vi "BiPotentiostat.vi"(4 "RE_Segments":i16[](array[numeric])=[0, 0, 0], 5 "AI Count(uSec)":u32=5, 6 "TE_Segments":i16[](array[numeric])=[0, 0, 0], 7 "Segment_uSec":sgl[](array[numeric])=[0.0, 0.0, 0.0], 8 "BE_Segments":i16[](array[numeric])=[0, 0, 0], 9 "RE_Start":i16, 10 "TE_Start":i16, 11 "BE_Start":i16) -> ()   [LabVIEW 2019]
uses:
  <vilib>/rvi/Emulation/niFpgaGetClockAttributes.vi
  <vilib>/rvi/Emulation/niFpgaSctlEmulationGetInTimedLoop.vi
  <vilib>/rvi/Emulation/niFpgaEmulationReportErrorSimple.vi
  <vilib>/rvi/eio/common/nirviEmuTemplateMethod_errors.vi
  <vilib>/rvi/interface/RandomDataEmulation/niFpgaRandomDataHandleErrors.vi
  <vilib>/rvi/Emulation/niFpgaProcessEmulError.vi
  <vilib>/rvi/DataTransferAndStorage/Container/Common/niFpgaContainerExecOnDevCompGetState.vi
  <vilib>/rvi/Emulation/niFpgaEmulationIsFPGAContextNoSignature.vi
  <vilib>/rvi/errors/niFpgaSetErrorForExecOnDevCompSimple.vi
  <vilib>/rvi/eio/common/nirviEmuReportErrorAndStop.vi
  <vilib>/rvi/DataTransferAndStorage/Container/Common/niFpgaContainerGetUniqueNameForEmu.vi
  <vilib>/rvi/FIFO/Fifo_Resource/nirvififoEmulationSetSize.vi
  <vilib>/rvi/FIFO/Fifo_Resource/nirviFifoEmulationQueueMgr.vi
  <instcachedir>/0/nirviFifoEmulationQueueMgr_E5CAEC123FF24DC58D834DCA3CDAA9B5.lvgen/nirviFifoEmulationQueueMgr_E5CAEC123FF24DC58D834DCA3CDAA9B5_008.vi
  <vilib>/rvi/FIFO/Fifo_Resource/nirvififoEmulationDetermineInputValidOut.vi
  <vilib>/rvi/FIFO/Fifo_Resource/nirvififoEmulationCreateLock.vi
  <vilib>/rvi/FIFO/Fifo_Resource/nirvififoEmulationObtainLock.vi
  <vilib>/rvi/FIFO/Fifo_Resource/nirvififoEmulationReleaseLock.vi
  <vilib>/rvi/occurrence/nirviWaitOnOccurrenceBase.vi
  <vilib>/rvi/errors/nirviReportUnexpectedCaseInternalError.vi
  <vilib>/rvi/errors/nirviReportUnexpectedCaseInternalError (U32).vi
  <vilib>/Utility/error.llb/Clear Errors.vi
  <vilib>/rvi/Emulation/niFpgaCriticalErrorInLSC.vi
  <vilib>/eio/EIONode/EIONode.xnode
  <vilib>/rvi/DataTransferAndStorage/Container/XNode/niFpgaContainer.xnode
  <vilib>/rvi/interface/RandomDataEmulation/nirviRandomDataFpgaReadWriteTemplate.vi
  <vilib>/rvi/FIFO/Fifo_Resource/niFpgaFifoEmulationRefIn.vi
panel:
  out "Stop":bool
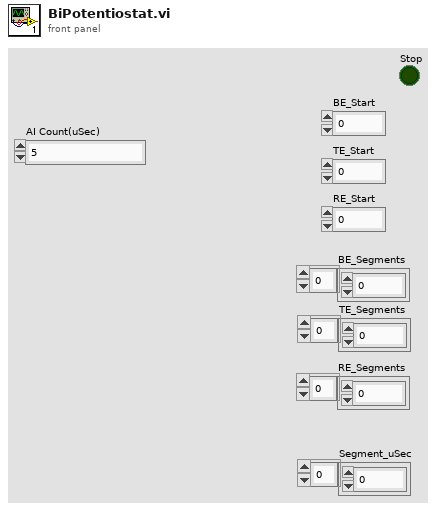
[diagram p1: front panel]
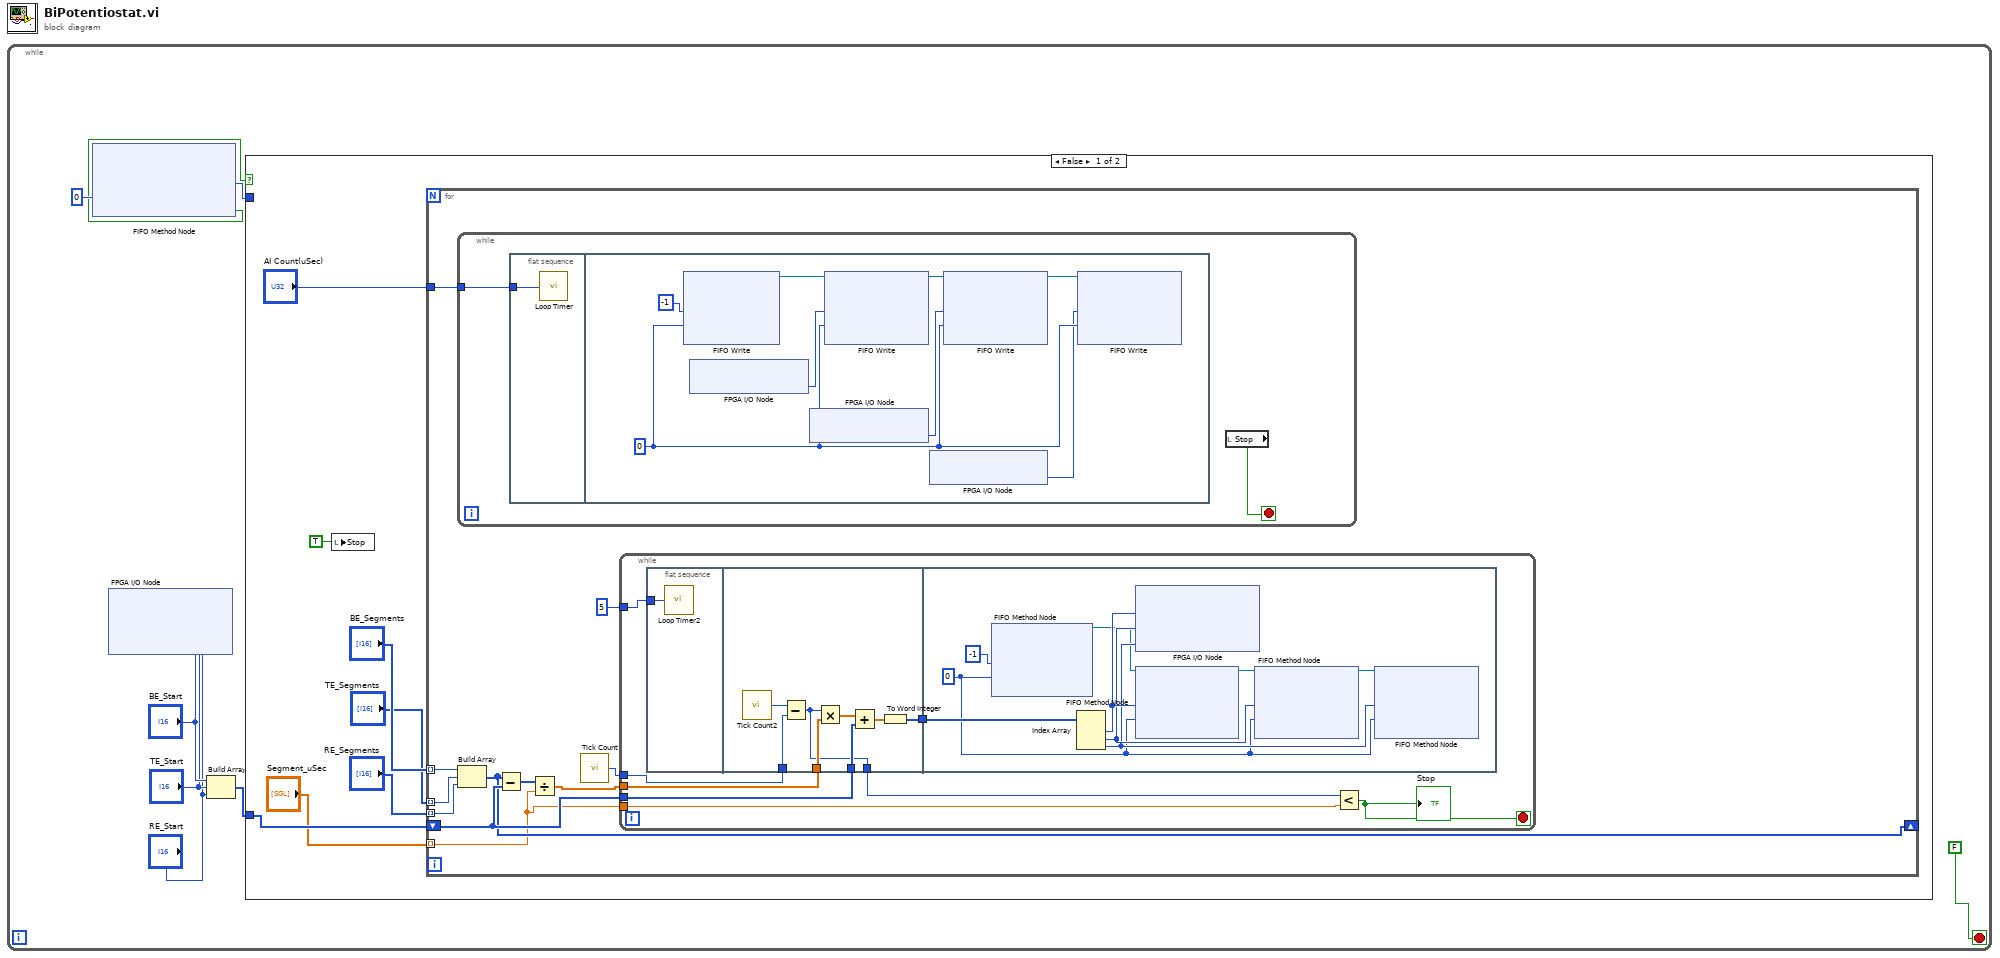
[diagram p0: block diagram]
diagram:
  n1 = while {
    stop <- FALSE stop-if-true
    n2 = xnode ("FIFO Method Node")("Timeout"=0) -> ("Element"=w6:i16, "Timed Out?"=w7:bool)  [unwired: 1 in, 1 out]
    n3 = xnode "FPGA I/O Node"("Connector0/AO0"="BE_Start", "Connector0/AO1"="TE_Start", "Connector0/AO2"="RE_Start") -> ()  [unwired: 3 in, 3 out]
    n4 = Build Array("BE_Start", "TE_Start", "RE_Start") -> (w1:i16[])
    n5 = case shown="False" w7 {
      tunnel: w6 -> [_ _]
      tunnel: w1 -> [w14 _]
      frame False {
        n6 = local write "Stop"(TRUE ("Stop")) -> ()
        n7 = for {
          tunnel: "AI Count(uSec)" -> [w26]
          shift-right: [w18] -> _
          shift-left: w14 -> [w19]
          tunnel: "Segment_uSec" -> [w16] mode=indexing
          tunnel: "BE_Segments" -> [w23] mode=indexing
          tunnel: "TE_Segments" -> [w22] mode=indexing
          tunnel: "RE_Segments" -> [w21] mode=indexing
          n8 = while {
            tunnel: w26 -> [w54]
            stop <- w53 stop-if-true
            n9 = flat-sequence {
              tunnel: w54 -> [w55]
              frame #0 {
                n10 = call "Loop Timer"("Count(uSec)"=w55) -> ()  [unwired: 1 out]
              }
              frame #1 {
                w60 = 0 ("Timeout")
                n11 = xnode ("FIFO Write")("Element"=i16 -1, "Timeout"=w60) -> ("FIFO Out"=w63:refnum<k21>)  [unwired: 1 in, 1 out]
                n12 = xnode "FPGA I/O Node"() -> ("Connector0/AI0"=w57:i16)  [unwired: 1 in, 1 out]
                n13 = xnode "FPGA I/O Node"() -> ("Connector0/AI1"=w58:i16)  [unwired: 1 in, 1 out]
                n14 = xnode ("FIFO Write")("Element"=w57, "Timeout"=w60, "FIFO In"=w63) -> ("FIFO Out"=w62:refnum<k21>)  [unwired: 1 out]
                n15 = xnode "FPGA I/O Node"() -> ("Connector0/AI2"=w59:i16)  [unwired: 1 in, 1 out]
                n16 = xnode ("FIFO Write")("Element"=w58, "Timeout"=w60, "FIFO In"=w62) -> ("FIFO Out"=w61:refnum<k21>)  [unwired: 1 out]
                n17 = xnode ("FIFO Write")("Element"=w59, "Timeout"=w60, "FIFO In"=w61) -> ()  [unwired: 2 out]
              }
            }
            n18 = local read "Stop"() -> (w53:bool)
          }
          n19 = Build Array(w23, w22, w21) -> (w18:i16[])
          n20 = Subtract(x=w18, y=w19) -> (x-y=w20:i16[])
          n21 = Divide(x=w20, y=w16) -> (x/y=w17:sgl[])
          n22 = call "Tick Count"() -> ("Tick Count(uSec)"=w24:u32)
          n23 = while {
            tunnel: u32 5 ("AO Count(uSec)") -> [w34]
            tunnel: w24 -> [w33]
            tunnel: w19 -> [w32]
            tunnel: w17 -> [w30]
            tunnel: w16 -> [w28]
            stop <- w27 stop-if-true
            n24 = flat-sequence {
              tunnel: w34 -> [w35]
              tunnel: w33 -> [w43]
              tunnel: w30 -> [w41]
              tunnel: w32 -> [w39]
              tunnel: [w37] -> w31
              tunnel: [w36] -> w29
              tunnel: w31 -> [w52]
              frame #0 {
                n25 = call "Loop Timer2"("Count(uSec)"=w35) -> ()  [unwired: 1 out]
              }
              frame #1 {
                n26 = call "Tick Count2"() -> ("Tick Count(uSec)"=w42:u32)
                n27 = Subtract(x=w42, y=w43) -> (x-y=w36:u32)
                n28 = Multiply(x=w36, y=w41) -> (x*y=w40:sgl[])
                n29 = Add(x=w40, y=w39) -> (x+y=w38:sgl[])
                n30 = To Word Integer(number=w38) -> (16bit integer=w37:i16[])
              }
              frame #2 {
                w47 = 0 ("Timeout")
                n31 = xnode ("FIFO Method Node")("Element"=i16 -1, "Timeout"=w47) -> ("FIFO Out"=w46:refnum<k21>)  [unwired: 1 in, 1 out]
                n32 = Index Array(array=w52) -> (element #1=w50:i16, element #2=w49:i16, element #3=w48:i16)  [unwired: 3 in]
                n33 = xnode "FPGA I/O Node"("Connector0/AO0"=w50, "Connector0/AO1"=w49, "Connector0/AO2"=w48) -> ()  [unwired: 3 in, 3 out]
                n34 = xnode ("FIFO Method Node")("Element"=w50, "Timeout"=w47, "FIFO In"=w46) -> ("FIFO Out"=w45:refnum<k21>)  [unwired: 1 out]
                n35 = xnode ("FIFO Method Node")("Element"=w49, "Timeout"=w47, "FIFO In"=w45) -> ("FIFO Out"=w44:refnum<k21>)  [unwired: 1 out]
                n36 = xnode ("FIFO Method Node")("Element"=w48, "Timeout"=w47, "FIFO In"=w44) -> ()  [unwired: 2 out]
              }
            }
            n37 = Less?(x=w29, y=w28) -> (x < y?=w27:bool)
            "Stop" <- w27
          }
        }
      }
      frame True {
      }
    }
  }
